vi "String Definition.vi"(11 "String in":refnum<class "String.lvclass">) -> (2 "Definition":T1={"Default"="", "Length"=255})   [LabVIEW 2020, in "Conditu2.lvlib" / "Columns.lvlib" / "String.lvclass"]
uses:
  String.lvclass
  Definition.ctl
  String.lvclass/String.ctl
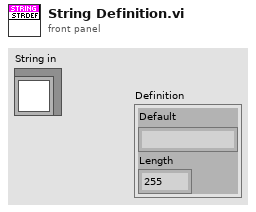
[diagram p1: front panel]
types:
  T1 = typedef "Conditu2.lvlib/Columns.lvlib/String.lvclass/Definition.ctl" = cluster{"Default":string, "Length":i32}
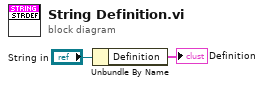
[diagram p0: block diagram]
diagram:
  n1 = Unbundle By Name("String in") -> ("Definition"=→"Definition":T1)
